vi "GUI_Single Button Pump.vi"() -> ()   [LabVIEW 2011] (continued)
        w1447 = T32[] [enum."Is the LB Roughing Pipe at Atmospheric Pressure?", enum."Is the LB Roughing Manifold at Atmospheric Pressure"] items=["No Action", "Is EC GPM Mode ON?", "Is EC GPM Mode Off?", "Is EC GVM Mode ON?", "Is EC GVM Off?", "Is  EC GPM or GVM Mode ON?", "Is LB GPM Mode ON?", "Is LB GPM Mode Off?", "Is LB GVM Mode ON?", "Is LB GVM Mode Off?", "Is  LB GPM or GVM Mode ON?", "Is M123 Turbo Gate Valve Opened? ", "Is M123 Turbo Gate Valve Closed?", "Is OAP Turbo Gate Valve Opened?", "Is OAP Turbo Gate Valve Closed?", "Is BTLTurbo Gate Valve Opened?", "Is BTL Turbo Gate Valve Closed?", "Is TARGET Turbo Gate Valve 1Opened?", "Is TARGET1 Turbo Gate Valve Closed?", "Is TARGET Turbo Gate Valve 2 Opened?", "Is TAREGT2 Turbo Gate Valve Closed?", "Is BTL2 Turbo Gate Valve Opened?", "Is BTL2 Turbo Gate Valve Closed?", "Is HPD Turbo Gate Valve Opened?", "Is HPD Turbo Gate Valve Closed?", "Is COMP to M123 gate Valve Opened?", "Is COMP to M123 Valve Closed?", "Is HPBD Gate Valve Opened?", "Is HPBD Gate Valve Closed?", "Is M123 to OAP gate valve opened?", "Is M123 to OAP gate valve closed?", "Is OAP to BLT gate valve opened?", "Is OAP to BTL Gate Valve Closed?", "Is BLT to TARGET gate valve opened?", "Is BTL to TARGET Gate Valve Closed?", "Is TARGET to BLT2 gate valve opened?", "Is TARGET to BTL2 Gate Valve Closed?", "Is BLT2 to HPD gate valve opened?", "Is BTL2 to HPD Gate Valve Closed?", "Is COMP at Atmospheric Pressure?", "Is M123 at Atmospheric Pressure?", "Is BeamDump at Atmospheric Pressure?", "Is OAP at Atmospheric Pressure?", "Is BLT at Atmospheric Pressure", "Is TARGET at Atmospheric Pressure?", "Is BLT2 at Atmospheric Pressure?", "Is HPD at Atmospheric Pressure?", "Is the EC Roughing Pump ON?", "Is the EC Roughing Pump OFF?", "Does the EC Roughing Pump have a fault?", "Is the LB Roughing Pump ON?", "Is the LB Roughing Pump Off?", "Does the LB Roughing Pump have a fault?", "Is the EC Backing Pump ON?", "Is the EC Backing Pump OFF?", "Is the LB Backing Pump ON?", "Is the LB Backing Pump OFF?", "Does the EC Backing Pump have a fault?", "Does the LB Backing Pump have a fault?", "Is the EC Backing Pipe at Atmospheric Pressure", "Is the LB Backing Pipe at Atmospheric Pressure", "Is the EC Backing Manifold at Atmospheric Pressure", "s the LB Backing Manifold at Atmospheric Pressure?", "Is the EC Roughing Pipe at Atmospheric Pressure", "Is the LB Roughing Pipe at Atmospheric Pressure?", "Is the EC Roughing Manifold at Atmospheric Pressure", "Is the LB Roughing Manifold at Atmospheric Pressure", "Is LB Backing Manifold Valve Opened?", "Is EC Backing Manifold Valve Opened?", "Is LB Roughing Manifold Valve Opened?", "Is EC Roughing Manifold Valve Opened?", "Is COMP Roughing Valve Opened?", "Is M123 Roughing Valve Opened?", "Is M123 Roughing Valve Closed?", "Is OAP Roughing Valve Opened?", "Is OAP Roughing Valve Closed?", "Is HPBD Roughing Valve Opened?", "Is HPBD Roughing Valve Closed?", "Is BTL Roughing Valve Opened?", "Is BTL Roughing Valve Closed?", "Is TARGET Roughing Valve Opened?", "Is TARGET Roughing Valve Closed?", "Is BTL2 Roughing Valve Opened?", "Is BTL2 Roughing Valve Closed?", "Is HPD Roughing Valve Opened?", "Is HPD Roughing Valve Closed?", "Is COMP Turbo Backing Valve Opened?", "Is M123 Turbo Backing Valve Opened", "Is HPBD Turbo Backing Valve Opened?", "Is OAP Turbo Backing Valve Opened?", "Is BTL Turbo Backing Valve Opened?", "Is TARGET1 Turbo Backing Valve Opened?", "Is TARGET2 Turbo Backing Valve Opened?", "Is BTL2 Turbo Backing Valve Opened?", "Is HPD Turbo Backing Valve Opened?", "Is M123 Backing at MID-VAC?", "Is OAP Backing at MID-VAC?", "Is TARGET1 Backing at MID-VAC?", "Is TARGET2 Backing at MID-VAC?", "Is BTL Backing at MID-VAC?", "Is BTL2 Backing at MID-VAC?", "Is HPD Backing at MID-VAC?", "Is M123 Turbo in Normal Operation", "Is COMP Turbo in Normal Operation", "Is OAP Turbo in Normal Operation", "Is BTL Turbo in Normal Operation", "Is TARGET1 Turbo in Normal Operation", "Is TARGET2 Turbo in Normal Operation", "Is BTL2 Turbo in Normal Operation", "Is HPD Turbo in Normal Operation", "Is M123 at MID-VAC?", "Is OAP at MID-VAC?", "Is COMP at MID-VAC?", "Is BTL at MID-VAC?", "Is TARGET at MID-VAC?", "Is BTL2 at MID-VAC?", "Is HPD at MID-VAC?"]
        # "Event TAG"
        n558 = Unbundle By Name(w1449) -> ("Chamber Selection"=w1448:T21)
        n559 = call "Selection ActionBuilder sections.vi"("EC Query Array"=w1446, "LB Query Array"=w1447, "Chamber Selection"=w1448) -> ("Query Array out"=w1445:T32[])  [unwired: 7 in, 1 out]
        n560 = call "GetAction.vi"("Check Condition"=w1462, "Query Array"=w1445, "input cluster"=w1449, "error in (no error)"=w1464) -> ("Status Array Out"=w1463:string[], "Generate Event?"=w1452:bool, "error out"=w1460:errorcluster)  [unwired: 6 in, 3 out]
        n561 = call "Generate User Event.vi"("Add(t)/Remove(f) Event"=w1452, "error in (no error)"=w1460, "User Event in"=w1461, "Status Array In"=w1463, "Error Codes"=w1462) -> ("error out"=w1459:errorcluster)  [unwired: 5 in, 1 out]
        n562 = Unbundle By Name(w1449) -> ("VI Refnum"=w1454:refnum<vi>)
        n563 = Not A Number/Path/Refnum?(number/path/refnum=w1454) -> (NaN/Path/Refnum?=w1453:bool)
        n564 = case shown="False" w1452 {
          tunnel: ["Main: Open Roughing Manifold Valves" w1480] -> w1450
          tunnel: w1454 -> [w1470 w1479]
          tunnel: w1453 -> [w1471 w1478]
          frame False {
            n565 = case shown="True" w1471 {
              tunnel: w1470 -> [_ w1474]
              frame False {
              }
              frame True {
                n566 = invoke class="VI" method="Abort VI"(reference=w1474) -> (reference out=w1472:refnum<vi>, error out=w1473:errorcluster)  [unwired: 2 in, 1 out]
                n567 = case shown="No Error" w1473 {
                  selector: w1473 -> [w1476 _]
                  tunnel: w1472 -> [w1477 _]
                  frame No Error {
                    n568 = Close Reference(reference=w1477, error in (no error)=w1476) -> (error out=w1475:errorcluster)
                    n569 = invoke on="User Input Panel" class="SubPnl" method="Remove VI"(error in=w1475) -> ()  [unwired: 2 in, 3 out]
                  }
                  frame Error {
                  }
                }
              }
            }
            n570 = call "MID-VAC Timer.vi"("TO sec (Start timer)"=5.0, "Action"=timerAction_typdef."Start Timer") -> ()  [unwired: 9 in, 1 out]
          }
          frame True {
            # "when to is true\nand"
            n571 = case shown="False" w1478 {
              tunnel: w1479 -> [w1484 _]
              tunnel: [w1482 "Main: Check Roughing Manifold Pressure Status"] -> w1480
              frame False {
                n572 = call "FindControlByName_VEPS.vi"("control name"="Op Out", "vi refnum"=w1484) -> ("control refnum"=w1486:refnum<vi>)  [unwired: 2 in, 1 out]
                n573 = property class="Ctl"(reference=w1486) -> ("Value"=w1485:variant)  [unwired: 1 in, 2 out]
                n574 = Variant To Data(type=op_typdef."Idle" ("Op Out"), Variant=w1485) -> (data=w1483:T24)  [unwired: 1 in, 1 out]
                n575 = case shown="\"Idle\", Default" w1483 {
                  tunnel: ["Main: Check Roughing Manifold Pressure Status" "Main: Check Roughing Manifold Pressure Status" "Idle\nMacro: Exit"] -> w1482
                  frame "Idle", Default {
                    n576 = call "MID-VAC Timer.vi"("TO sec (Start timer)"=30.0, "Action"=timerAction_typdef."Start Timer") -> ()  [unwired: 9 in, 1 out]
                  }
                  frame "Continue to Wait" {
                    # "Continue to wait. Reset Timer"
                    n577 = call "MID-VAC Timer.vi"("TO sec (Start timer)"=30.0, "Action"=timerAction_typdef."Start Timer") -> ()  [unwired: 9 in, 1 out]
                  }
                  frame "Exit" {
                  }
                }
              }
              frame True {
              }
            }
          }
        }
        n578 = call "MID-VAC Timer.vi"("Action"=timerAction_typdef."Timer Running") -> ("TO"=w1457:bool)  [unwired: 10 in]
        n579 = And(x=w1452, y=w1457) -> (x .and. y?=w1456:bool)
        n580 = call "Generate TO event.vi"("Boolean"=w1456, "message"="Roughing Pipe and Manifold are not Vented\nPlease perform corrective action\n and click on continue.\nClick Exit to abort GPM", "User Event in"=w1451) -> ()  [unwired: 9 in]
        n581 = call <vilib>:"Add State(s) to Queue__jki_lib_state_machine.vi"("State(s) in (\"\")"=w1466, "State(s) at Back (\"\")"=w1450) -> ("States Out"=w1465:string)  [unwired: 13 in]
      }
      frame "Main: Open Roughing Manifold Valves" {
        # "Open Backing Valves on both systems"
        n582 = Unbundle By Name(w1497) -> ("Debug Mode?"=w1496:bool)
        n583 = case shown="False" w1496 {
          tunnel: w1503 -> [w1513 w1518]
          tunnel: [w1510 w1518] -> w1501
          tunnel: w1497 -> [w1508 _]
          frame False {
            w1507 = T33[] [enum."Open LB Roughing Valve"] items=["No Action", "Set GPM Mode LB", "EXIT GPM Mode LB", "Set GPM Mode EC", "EXIT GPM Mode EC", "Set GVM mode LB", "Set GVM Mode EC", "Open LB Backing Valve", "Open EC Backing Valve", "Open EC Roughing Valve", "Open LB Roughing Valve", "Open M123 Roughing Valve", "Close M123 Roughing Valve", "Open Compressor Roughing Valve", "Close Compressor Roughing Valve", "Open BeamDump Roughing Valve", "Close BeamDump Roughing Valve", "Open OAP Roughing Valve", "Close OAP Roughing Valve", "Open BTL Roughing Valve", "Close BTL Roughing Valve", "Open Target Roughing Valve", "Close Target Roughing Valve", "Open BTL2 Roughing Valve", "Close BTL2 Roughing Valve", "Open HPD Roughing Valve", "Close HPD Roughing Valve", "LB Start Roughing Pump ", "EC Start Roughing Pump", "Open COMP Turbo Backing Valve", "Open M123 Turbo Backing Valve", "Open OAP Turbo Backing Valve", "Open HPBD Turbo Backing Valve", "Open BLT Turbo Backing Valve", "Open TARGET1 Turbo Backing Valve", "Open TARGET2 Turbo Backing Valve", "Open BLT2 Turbo Backing Valve", "Open HPD Turbo Backing Valve", "LB Start Turbo Backing Pump", "EC Start Turbo Backing Pump", "Start COMP Turbo Pump", "Start M123 Turbo Pump", "Start OAP Turbo Pump", "Start BTL Turbo Pump", "Start TARGET1 Turbo Pump", "Start TARGET2 Turbo Pump", "Start BTL2 Turbo Pump", "Start HPD Turbo Pump", "Open COMP Turbo Gate Valve", "Open M123 Turbo Gate Valve", "Open OAP Turbo Gate Valve", "Open BTL Turbo Gate Valve", "Open TARGET1 Turbo Gate Valve", "Open TARGET2 Turbo Gate Valve", "Open BTL2 Turbo Gate Valve", "Open HPD Turbo Gate Valve"]
            w1506 = T33[] [enum."Open EC Roughing Valve"] items=["No Action", "Set GPM Mode LB", "EXIT GPM Mode LB", "Set GPM Mode EC", "EXIT GPM Mode EC", "Set GVM mode LB", "Set GVM Mode EC", "Open LB Backing Valve", "Open EC Backing Valve", "Open EC Roughing Valve", "Open LB Roughing Valve", "Open M123 Roughing Valve", "Close M123 Roughing Valve", "Open Compressor Roughing Valve", "Close Compressor Roughing Valve", "Open BeamDump Roughing Valve", "Close BeamDump Roughing Valve", "Open OAP Roughing Valve", "Close OAP Roughing Valve", "Open BTL Roughing Valve", "Close BTL Roughing Valve", "Open Target Roughing Valve", "Close Target Roughing Valve", "Open BTL2 Roughing Valve", "Close BTL2 Roughing Valve", "Open HPD Roughing Valve", "Close HPD Roughing Valve", "LB Start Roughing Pump ", "EC Start Roughing Pump", "Open COMP Turbo Backing Valve", "Open M123 Turbo Backing Valve", "Open OAP Turbo Backing Valve", "Open HPBD Turbo Backing Valve", "Open BLT Turbo Backing Valve", "Open TARGET1 Turbo Backing Valve", "Open TARGET2 Turbo Backing Valve", "Open BLT2 Turbo Backing Valve", "Open HPD Turbo Backing Valve", "LB Start Turbo Backing Pump", "EC Start Turbo Backing Pump", "Start COMP Turbo Pump", "Start M123 Turbo Pump", "Start OAP Turbo Pump", "Start BTL Turbo Pump", "Start TARGET1 Turbo Pump", "Start TARGET2 Turbo Pump", "Start BTL2 Turbo Pump", "Start HPD Turbo Pump", "Open COMP Turbo Gate Valve", "Open M123 Turbo Gate Valve", "Open OAP Turbo Gate Valve", "Open BTL Turbo Gate Valve", "Open TARGET1 Turbo Gate Valve", "Open TARGET2 Turbo Gate Valve", "Open BTL2 Turbo Gate Valve", "Open HPD Turbo Gate Valve"]
            n584 = Unbundle By Name(w1508) -> ("Chamber Selection"=w1509:T21)
            n585 = call "Selection ActionBuilder sections.vi"("EC Command Array"=w1506, "Chamber Selection"=w1509, "LB Command Array"=w1507) -> ("Command Array out"=w1505:T33[])  [unwired: 7 in, 1 out]
            n586 = Unbundle By Name(w1508) -> ("TCPConnection.Command TCP Connection EC"=w1514:refnum<k5>)
            n587 = Unbundle By Name(w1508) -> ("TCPConnection.Command TCP Connection LB"=w1516:refnum<k5>)
            n588 = call "Build Command.vi"("Command Array in"=w1505, "input cluster"=w1508) -> ("output EC Command cluster"=w1515:T34, "output LB Command cluster"=w1517:T34)  [unwired: 8 in]
            n589 = call "Send Command LB.vi"("error in (no error)"=w1513, "output LB Command cluster"=w1517, "TCP Network Connection in"=w1516) -> ("error out"=w1511:errorcluster)  [unwired: 8 in]
            n590 = call "Send Command EC.vi"("error in (no error)"=w1513, "output EC Command cluster"=w1515, "TCP Network Connection in"=w1514) -> ("error out"=w1512:errorcluster)  [unwired: 8 in]
            n591 = Merge Errors(w1511, w1512) -> (w1510:errorcluster)
          }
          frame True {
          }
        }
        n592 = call "Reset Command Clusters.vi"("error in (no error)"=w1501, "input cluster"=w1497) -> ("error out"=w1500:errorcluster, "output cluster"=w1499:T20)  [unwired: 8 in]
        n593 = call <vilib>:"Add State(s) to Queue__jki_lib_state_machine.vi"("State(s) in Front (\"\")"="Main: Check Roughing Manifold Valve Status", "State(s) in (\"\")"=w1498) -> ("States Out"=w1504:string)  [unwired: 13 in]
      }
      frame "Main: Check Roughing Manifold Valve Status" {
        w1521 = T32[] [enum."Is EC Roughing Manifold Valve Opened?"] items=["No Action", "Is EC GPM Mode ON?", "Is EC GPM Mode Off?", "Is EC GVM Mode ON?", "Is EC GVM Off?", "Is  EC GPM or GVM Mode ON?", "Is LB GPM Mode ON?", "Is LB GPM Mode Off?", "Is LB GVM Mode ON?", "Is LB GVM Mode Off?", "Is  LB GPM or GVM Mode ON?", "Is M123 Turbo Gate Valve Opened? ", "Is M123 Turbo Gate Valve Closed?", "Is OAP Turbo Gate Valve Opened?", "Is OAP Turbo Gate Valve Closed?", "Is BTLTurbo Gate Valve Opened?", "Is BTL Turbo Gate Valve Closed?", "Is TARGET Turbo Gate Valve 1Opened?", "Is TARGET1 Turbo Gate Valve Closed?", "Is TARGET Turbo Gate Valve 2 Opened?", "Is TAREGT2 Turbo Gate Valve Closed?", "Is BTL2 Turbo Gate Valve Opened?", "Is BTL2 Turbo Gate Valve Closed?", "Is HPD Turbo Gate Valve Opened?", "Is HPD Turbo Gate Valve Closed?", "Is COMP to M123 gate Valve Opened?", "Is COMP to M123 Valve Closed?", "Is HPBD Gate Valve Opened?", "Is HPBD Gate Valve Closed?", "Is M123 to OAP gate valve opened?", "Is M123 to OAP gate valve closed?", "Is OAP to BLT gate valve opened?", "Is OAP to BTL Gate Valve Closed?", "Is BLT to TARGET gate valve opened?", "Is BTL to TARGET Gate Valve Closed?", "Is TARGET to BLT2 gate valve opened?", "Is TARGET to BTL2 Gate Valve Closed?", "Is BLT2 to HPD gate valve opened?", "Is BTL2 to HPD Gate Valve Closed?", "Is COMP at Atmospheric Pressure?", "Is M123 at Atmospheric Pressure?", "Is BeamDump at Atmospheric Pressure?", "Is OAP at Atmospheric Pressure?", "Is BLT at Atmospheric Pressure", "Is TARGET at Atmospheric Pressure?", "Is BLT2 at Atmospheric Pressure?", "Is HPD at Atmospheric Pressure?", "Is the EC Roughing Pump ON?", "Is the EC Roughing Pump OFF?", "Does the EC Roughing Pump have a fault?", "Is the LB Roughing Pump ON?", "Is the LB Roughing Pump Off?", "Does the LB Roughing Pump have a fault?", "Is the EC Backing Pump ON?", "Is the EC Backing Pump OFF?", "Is the LB Backing Pump ON?", "Is the LB Backing Pump OFF?", "Does the EC Backing Pump have a fault?", "Does the LB Backing Pump have a fault?", "Is the EC Backing Pipe at Atmospheric Pressure", "Is the LB Backing Pipe at Atmospheric Pressure", "Is the EC Backing Manifold at Atmospheric Pressure", "s the LB Backing Manifold at Atmospheric Pressure?", "Is the EC Roughing Pipe at Atmospheric Pressure", "Is the LB Roughing Pipe at Atmospheric Pressure?", "Is the EC Roughing Manifold at Atmospheric Pressure", "Is the LB Roughing Manifold at Atmospheric Pressure", "Is LB Backing Manifold Valve Opened?", "Is EC Backing Manifold Valve Opened?", "Is LB Roughing Manifold Valve Opened?", "Is EC Roughing Manifold Valve Opened?", "Is COMP Roughing Valve Opened?", "Is M123 Roughing Valve Opened?", "Is M123 Roughing Valve Closed?", "Is OAP Roughing Valve Opened?", "Is OAP Roughing Valve Closed?", "Is HPBD Roughing Valve Opened?", "Is HPBD Roughing Valve Closed?", "Is BTL Roughing Valve Opened?", "Is BTL Roughing Valve Closed?", "Is TARGET Roughing Valve Opened?", "Is TARGET Roughing Valve Closed?", "Is BTL2 Roughing Valve Opened?", "Is BTL2 Roughing Valve Closed?", "Is HPD Roughing Valve Opened?", "Is HPD Roughing Valve Closed?", "Is COMP Turbo Backing Valve Opened?", "Is M123 Turbo Backing Valve Opened", "Is HPBD Turbo Backing Valve Opened?", "Is OAP Turbo Backing Valve Opened?", "Is BTL Turbo Backing Valve Opened?", "Is TARGET1 Turbo Backing Valve Opened?", "Is TARGET2 Turbo Backing Valve Opened?", "Is BTL2 Turbo Backing Valve Opened?", "Is HPD Turbo Backing Valve Opened?", "Is M123 Backing at MID-VAC?", "Is OAP Backing at MID-VAC?", "Is TARGET1 Backing at MID-VAC?", "Is TARGET2 Backing at MID-VAC?", "Is BTL Backing at MID-VAC?", "Is BTL2 Backing at MID-VAC?", "Is HPD Backing at MID-VAC?", "Is M123 Turbo in Normal Operation", "Is COMP Turbo in Normal Operation", "Is OAP Turbo in Normal Operation", "Is BTL Turbo in Normal Operation", "Is TARGET1 Turbo in Normal Operation", "Is TARGET2 Turbo in Normal Operation", "Is BTL2 Turbo in Normal Operation", "Is HPD Turbo in Normal Operation", "Is M123 at MID-VAC?", "Is OAP at MID-VAC?", "Is COMP at MID-VAC?", "Is BTL at MID-VAC?", "Is TARGET at MID-VAC?", "Is BTL2 at MID-VAC?", "Is HPD at MID-VAC?"]
        w1536 = Error_codes."010-Roughing Valve Status" ("Error Codes")
        w1520 = T32[] [enum."Is LB Roughing Manifold Valve Opened?"] items=["No Action", "Is EC GPM Mode ON?", "Is EC GPM Mode Off?", "Is EC GVM Mode ON?", "Is EC GVM Off?", "Is  EC GPM or GVM Mode ON?", "Is LB GPM Mode ON?", "Is LB GPM Mode Off?", "Is LB GVM Mode ON?", "Is LB GVM Mode Off?", "Is  LB GPM or GVM Mode ON?", "Is M123 Turbo Gate Valve Opened? ", "Is M123 Turbo Gate Valve Closed?", "Is OAP Turbo Gate Valve Opened?", "Is OAP Turbo Gate Valve Closed?", "Is BTLTurbo Gate Valve Opened?", "Is BTL Turbo Gate Valve Closed?", "Is TARGET Turbo Gate Valve 1Opened?", "Is TARGET1 Turbo Gate Valve Closed?", "Is TARGET Turbo Gate Valve 2 Opened?", "Is TAREGT2 Turbo Gate Valve Closed?", "Is BTL2 Turbo Gate Valve Opened?", "Is BTL2 Turbo Gate Valve Closed?", "Is HPD Turbo Gate Valve Opened?", "Is HPD Turbo Gate Valve Closed?", "Is COMP to M123 gate Valve Opened?", "Is COMP to M123 Valve Closed?", "Is HPBD Gate Valve Opened?", "Is HPBD Gate Valve Closed?", "Is M123 to OAP gate valve opened?", "Is M123 to OAP gate valve closed?", "Is OAP to BLT gate valve opened?", "Is OAP to BTL Gate Valve Closed?", "Is BLT to TARGET gate valve opened?", "Is BTL to TARGET Gate Valve Closed?", "Is TARGET to BLT2 gate valve opened?", "Is TARGET to BTL2 Gate Valve Closed?", "Is BLT2 to HPD gate valve opened?", "Is BTL2 to HPD Gate Valve Closed?", "Is COMP at Atmospheric Pressure?", "Is M123 at Atmospheric Pressure?", "Is BeamDump at Atmospheric Pressure?", "Is OAP at Atmospheric Pressure?", "Is BLT at Atmospheric Pressure", "Is TARGET at Atmospheric Pressure?", "Is BLT2 at Atmospheric Pressure?", "Is HPD at Atmospheric Pressure?", "Is the EC Roughing Pump ON?", "Is the EC Roughing Pump OFF?", "Does the EC Roughing Pump have a fault?", "Is the LB Roughing Pump ON?", "Is the LB Roughing Pump Off?", "Does the LB Roughing Pump have a fault?", "Is the EC Backing Pump ON?", "Is the EC Backing Pump OFF?", "Is the LB Backing Pump ON?", "Is the LB Backing Pump OFF?", "Does the EC Backing Pump have a fault?", "Does the LB Backing Pump have a fault?", "Is the EC Backing Pipe at Atmospheric Pressure", "Is the LB Backing Pipe at Atmospheric Pressure", "Is the EC Backing Manifold at Atmospheric Pressure", "s the LB Backing Manifold at Atmospheric Pressure?", "Is the EC Roughing Pipe at Atmospheric Pressure", "Is the LB Roughing Pipe at Atmospheric Pressure?", "Is the EC Roughing Manifold at Atmospheric Pressure", "Is the LB Roughing Manifold at Atmospheric Pressure", "Is LB Backing Manifold Valve Opened?", "Is EC Backing Manifold Valve Opened?", "Is LB Roughing Manifold Valve Opened?", "Is EC Roughing Manifold Valve Opened?", "Is COMP Roughing Valve Opened?", "Is M123 Roughing Valve Opened?", "Is M123 Roughing Valve Closed?", "Is OAP Roughing Valve Opened?", "Is OAP Roughing Valve Closed?", "Is HPBD Roughing Valve Opened?", "Is HPBD Roughing Valve Closed?", "Is BTL Roughing Valve Opened?", "Is BTL Roughing Valve Closed?", "Is TARGET Roughing Valve Opened?", "Is TARGET Roughing Valve Closed?", "Is BTL2 Roughing Valve Opened?", "Is BTL2 Roughing Valve Closed?", "Is HPD Roughing Valve Opened?", "Is HPD Roughing Valve Closed?", "Is COMP Turbo Backing Valve Opened?", "Is M123 Turbo Backing Valve Opened", "Is HPBD Turbo Backing Valve Opened?", "Is OAP Turbo Backing Valve Opened?", "Is BTL Turbo Backing Valve Opened?", "Is TARGET1 Turbo Backing Valve Opened?", "Is TARGET2 Turbo Backing Valve Opened?", "Is BTL2 Turbo Backing Valve Opened?", "Is HPD Turbo Backing Valve Opened?", "Is M123 Backing at MID-VAC?", "Is OAP Backing at MID-VAC?", "Is TARGET1 Backing at MID-VAC?", "Is TARGET2 Backing at MID-VAC?", "Is BTL Backing at MID-VAC?", "Is BTL2 Backing at MID-VAC?", "Is HPD Backing at MID-VAC?", "Is M123 Turbo in Normal Operation", "Is COMP Turbo in Normal Operation", "Is OAP Turbo in Normal Operation", "Is BTL Turbo in Normal Operation", "Is TARGET1 Turbo in Normal Operation", "Is TARGET2 Turbo in Normal Operation", "Is BTL2 Turbo in Normal Operation", "Is HPD Turbo in Normal Operation", "Is M123 at MID-VAC?", "Is OAP at MID-VAC?", "Is COMP at MID-VAC?", "Is BTL at MID-VAC?", "Is TARGET at MID-VAC?", "Is BTL2 at MID-VAC?", "Is HPD at MID-VAC?"]
        # "Event TAG"
        n594 = Unbundle By Name(w1522) -> ("Chamber Selection"=w1523:T21)
        n595 = call "Selection ActionBuilder sections.vi"("EC Query Array"=w1521, "LB Query Array"=w1520, "Chamber Selection"=w1523) -> ("Query Array out"=w1519:T32[])  [unwired: 7 in, 1 out]
        n596 = call "GetAction.vi"("Check Condition"=w1536, "Query Array"=w1519, "input cluster"=w1522, "error in (no error)"=w1538) -> ("Status Array Out"=w1537:string[], "Generate Event?"=w1526:bool, "error out"=w1534:errorcluster)  [unwired: 6 in, 3 out]
        n597 = call "Generate User Event.vi"("Add(t)/Remove(f) Event"=w1526, "error in (no error)"=w1534, "User Event in"=w1535, "Status Array In"=w1537, "Error Codes"=w1536) -> ("error out"=w1533:errorcluster)  [unwired: 5 in, 1 out]
        n598 = Unbundle By Name(w1522) -> ("VI Refnum"=w1528:refnum<vi>)
        n599 = Not A Number/Path/Refnum?(number/path/refnum=w1528) -> (NaN/Path/Refnum?=w1527:bool)
        n600 = case shown="False" w1526 {
          tunnel: ["Macro: Roughing Valve Precheck Selection" w1554] -> w1524
          tunnel: w1528 -> [w1544 w1553]
          tunnel: w1527 -> [w1545 w1552]
          frame False {
            # "Proceed to next step"
            n601 = case shown="False" w1545 {
              tunnel: w1544 -> [_ w1548]
              frame False {
              }
              frame True {
                n602 = invoke class="VI" method="Abort VI"(reference=w1548) -> (reference out=w1546:refnum<vi>, error out=w1547:errorcluster)  [unwired: 2 in, 1 out]
                n603 = case shown="No Error" w1547 {
                  selector: w1547 -> [w1550 _]
                  tunnel: w1546 -> [w1551 _]
                  frame No Error {
                    n604 = Close Reference(reference=w1551, error in (no error)=w1550) -> (error out=w1549:errorcluster)
                    n605 = invoke on="User Input Panel" class="SubPnl" method="Remove VI"(error in=w1549) -> ()  [unwired: 2 in, 3 out]
                  }
                  frame Error {
                  }
                }
              }
            }
            n606 = call "MID-VAC Timer.vi"("TO sec (Start timer)"=5.0, "Action"=timerAction_typdef."Start Timer") -> ()  [unwired: 9 in, 1 out]
          }
          frame True {
            # "when to is true\nand"
            n607 = case shown="False" w1552 {
              tunnel: w1553 -> [w1558 _]
              tunnel: [w1556 "Main: Check Roughing Manifold Valve Status"] -> w1554
              frame False {
                n608 = call "FindControlByName_VEPS.vi"("control name"="Op Out", "vi refnum"=w1558) -> ("control refnum"=w1560:refnum<vi>)  [unwired: 2 in, 1 out]
                n609 = property class="Ctl"(reference=w1560) -> ("Value"=w1559:variant)  [unwired: 1 in, 2 out]
                n610 = Variant To Data(type=op_typdef."Idle" ("Op Out"), Variant=w1559) -> (data=w1557:T24)  [unwired: 1 in, 1 out]
                n611 = case shown="\"Idle\", Default" w1557 {
                  tunnel: ["Main: Check Roughing Manifold Valve Status" "Main: Check Roughing Manifold Valve Status" "Idle\nMacro: Exit"] -> w1556
                  frame "Idle", Default {
                    n612 = call "MID-VAC Timer.vi"("TO sec (Start timer)"=30.0, "Action"=timerAction_typdef."Start Timer") -> ()  [unwired: 9 in, 1 out]
                  }
                  frame "Continue to Wait" {
                    # "Continue to wait. Reset Timer"
                    n613 = call "MID-VAC Timer.vi"("TO sec (Start timer)"=30.0, "Action"=timerAction_typdef."Start Timer") -> ()  [unwired: 9 in, 1 out]
                  }
                  frame "Exit" {
                  }
                }
              }
              frame True {
              }
            }
          }
        }
        n614 = call "MID-VAC Timer.vi"("Action"=timerAction_typdef."Timer Running") -> ("TO"=w1531:bool)  [unwired: 10 in]
        n615 = And(x=w1526, y=w1531) -> (x .and. y?=w1530:bool)
        n616 = call <vilib>:"Add State(s) to Queue__jki_lib_state_machine.vi"("State(s) in Front (\"\")"=w1524, "State(s) in (\"\")"=w1540) -> ("States Out"=w1539:string)  [unwired: 13 in]
        n617 = call "Generate TO event.vi"("Boolean"=w1530, "message"="Roughing Manifold Valve is NOT open.\nPlease perform corrective action\nClick on continue to wait for 30 seconds.\nClick Exit to abort GPM", "User Event in"=w1525) -> ()  [unwired: 9 in]
      }
      frame "---------- Main: Roughing Valves----------" {
      }
      frame "Macro: Roughing Valve Precheck Selection" {
        # "3. Start Roughing pumps after all prechecks for roughing valves\nhave been completed and the roughing valves for selected chambers\nare opened."
        # "1. Check if only some chambers are selected"
        n618 = Unbundle By Name(w1578) -> ("Chamber Selection"=w1577:T21, "Isolate HPBD"=w1580:bool, "GPM Mode"=w1582:T1)
        n619 = Equal?(x=w1582, y=GPM_Mode_typdef."Complete Global Pump Mode" ("GPM Mode")) -> (x = y?=w1579:bool)
        n620 = case shown="True" w1579 {
          tunnel: [w1586 w1590] -> w1574
          tunnel: w1580 -> [w1588 w1589]
          tunnel: w1578 -> [_ _]
          tunnel: w1577 -> [w1587 _]
          frame False {
            # "2. All chambers not selected. Roughing Valve checks \nwill be performed only on selected chambers"
            n621 = call "Roughing Valve Precheck Selection.vi"("Isolate HPBD"=w1588, "Chamber Selection"=w1587) -> ("States Out"=w1586:string)  [unwired: 9 in]
          }
          frame True {
            # "2. All chambers are selected."
            n622 = case shown="False" w1589 {
              tunnel: ["Main: Roughing Valve Precheck>>M123\nMain: Open Roughing Valve>>M123\nMain: Check Roughing Valve Status>>M123\nMain: Roughing Valve Precheck>>HPBD\nMain: Open Roughing Valve>>HPBD\nMain: Check Roughing Valve Status>>HPBD\nMain: Roughing Valve Precheck>>OAP\nMain: Open Roughing Valve>>OAP\nMain: Check Roughing Valve Status>>OAP\nMain: Roughing Valve Precheck>>BTL\nMain: Open Roughing Valve>>BTL\nMain: Check Roughing Valve Status>>BTL\nMain: Roughing Valve Precheck>>TARGET\nMain: Open Roughing Valve>>TARGET\nMain: Check Roughing Valve Status>>TARGET\nMain: Roughing Valve Precheck>>BTL2\nMain: Open Roughing Valve>>BTL2\nMain: Check Roughing Valve Status>>BTL2\nMain: Roughing Valve Precheck>>HPD\nMain: Open Roughing Valve>>HPD\nMain: Check Roughing Valve Status>>HPD" "Main: Roughing Valve Precheck>>M123\nMain: Open Roughing Valve>>M123\nMain: Check Roughing Valve Status>>M123\nMain: Roughing Valve Precheck>>OAP\nMain: Open Roughing Valve>>OAP\nMain: Check Roughing Valve Status>>OAP\nMain: Roughing Valve Precheck>>BTL\nMain: Open Roughing Valve>>BTL\nMain: Check Roughing Valve Status>>BTL\nMain: Roughing Valve Precheck>>TARGET\nMain: Open Roughing Valve>>TARGET\nMain: Check Roughing Valve Status>>TARGET\nMain: Roughing Valve Precheck>>BTL2\nMain: Open Roughing Valve>>BTL2\nMain: Check Roughing Valve Status>>BTL2\nMain: Roughing Valve Precheck>>HPD\nMain: Open Roughing Valve>>HPD\nMain: Check Roughing Valve Status>>HPD"] -> w1590
              frame False {
                # "HPBD is NOT Isolated"
              }
              frame True {
                # "HPBD is Isolated"
              }
            }
          }
        }
        n623 = Concatenate Strings(w1574, "\n", "Main: Start Roughing Pumps" ("string")) -> (w1573:string)
        n624 = call <vilib>:"Add State(s) to Queue__jki_lib_state_machine.vi"("State(s) in Front (\"\")"=w1573, "State(s) in (\"\")"=w1585) -> ("States Out"=w1584:string)  [unwired: 13 in]
      }
      frame "Main: Roughing Valve Precheck" {
        w1606 = Error_codes."004-Check Chamber Pressures" ("Error Codes")
        n625 = case shown="\"BTL2\"" w1596 {
          tunnel: [_ w1630 w1631 w1632 w1633 w1634 w1635 w1636] -> w1609
          frame "False", Default {
          }
          frame "M123" {
            w1630 = T32[] [enum."Is M123 at Atmospheric Pressure?", enum."Is the LB Roughing Manifold at Atmospheric Pressure"] items=["No Action", "Is EC GPM Mode ON?", "Is EC GPM Mode Off?", "Is EC GVM Mode ON?", "Is EC GVM Off?", "Is  EC GPM or GVM Mode ON?", "Is LB GPM Mode ON?", "Is LB GPM Mode Off?", "Is LB GVM Mode ON?", "Is LB GVM Mode Off?", "Is  LB GPM or GVM Mode ON?", "Is M123 Turbo Gate Valve Opened? ", "Is M123 Turbo Gate Valve Closed?", "Is OAP Turbo Gate Valve Opened?", "Is OAP Turbo Gate Valve Closed?", "Is BTLTurbo Gate Valve Opened?", "Is BTL Turbo Gate Valve Closed?", "Is TARGET Turbo Gate Valve 1Opened?", "Is TARGET1 Turbo Gate Valve Closed?", "Is TARGET Turbo Gate Valve 2 Opened?", "Is TAREGT2 Turbo Gate Valve Closed?", "Is BTL2 Turbo Gate Valve Opened?", "Is BTL2 Turbo Gate Valve Closed?", "Is HPD Turbo Gate Valve Opened?", "Is HPD Turbo Gate Valve Closed?", "Is COMP to M123 gate Valve Opened?", "Is COMP to M123 Valve Closed?", "Is HPBD Gate Valve Opened?", "Is HPBD Gate Valve Closed?", "Is M123 to OAP gate valve opened?", "Is M123 to OAP gate valve closed?", "Is OAP to BLT gate valve opened?", "Is OAP to BTL Gate Valve Closed?", "Is BLT to TARGET gate valve opened?", "Is BTL to TARGET Gate Valve Closed?", "Is TARGET to BLT2 gate valve opened?", "Is TARGET to BTL2 Gate Valve Closed?", "Is BLT2 to HPD gate valve opened?", "Is BTL2 to HPD Gate Valve Closed?", "Is COMP at Atmospheric Pressure?", "Is M123 at Atmospheric Pressure?", "Is BeamDump at Atmospheric Pressure?", "Is OAP at Atmospheric Pressure?", "Is BLT at Atmospheric Pressure", "Is TARGET at Atmospheric Pressure?", "Is BLT2 at Atmospheric Pressure?", "Is HPD at Atmospheric Pressure?", "Is the EC Roughing Pump ON?", "Is the EC Roughing Pump OFF?", "Does the EC Roughing Pump have a fault?", "Is the LB Roughing Pump ON?", "Is the LB Roughing Pump Off?", "Does the LB Roughing Pump have a fault?", "Is the EC Backing Pump ON?", "Is the EC Backing Pump OFF?", "Is the LB Backing Pump ON?", "Is the LB Backing Pump OFF?", "Does the EC Backing Pump have a fault?", "Does the LB Backing Pump have a fault?", "Is the EC Backing Pipe at Atmospheric Pressure", "Is the LB Backing Pipe at Atmospheric Pressure", "Is the EC Backing Manifold at Atmospheric Pressure", "s the LB Backing Manifold at Atmospheric Pressure?", "Is the EC Roughing Pipe at Atmospheric Pressure", "Is the LB Roughing Pipe at Atmospheric Pressure?", "Is the EC Roughing Manifold at Atmospheric Pressure", "Is the LB Roughing Manifold at Atmospheric Pressure", "Is LB Backing Manifold Valve Opened?", "Is EC Backing Manifold Valve Opened?", "Is LB Roughing Manifold Valve Opened?", "Is EC Roughing Manifold Valve Opened?", "Is COMP Roughing Valve Opened?", "Is M123 Roughing Valve Opened?", "Is M123 Roughing Valve Closed?", "Is OAP Roughing Valve Opened?", "Is OAP Roughing Valve Closed?", "Is HPBD Roughing Valve Opened?", "Is HPBD Roughing Valve Closed?", "Is BTL Roughing Valve Opened?", "Is BTL Roughing Valve Closed?", "Is TARGET Roughing Valve Opened?", "Is TARGET Roughing Valve Closed?", "Is BTL2 Roughing Valve Opened?", "Is BTL2 Roughing Valve Closed?", "Is HPD Roughing Valve Opened?", "Is HPD Roughing Valve Closed?", "Is COMP Turbo Backing Valve Opened?", "Is M123 Turbo Backing Valve Opened", "Is HPBD Turbo Backing Valve Opened?", "Is OAP Turbo Backing Valve Opened?", "Is BTL Turbo Backing Valve Opened?", "Is TARGET1 Turbo Backing Valve Opened?", "Is TARGET2 Turbo Backing Valve Opened?", "Is BTL2 Turbo Backing Valve Opened?", "Is HPD Turbo Backing Valve Opened?", "Is M123 Backing at MID-VAC?", "Is OAP Backing at MID-VAC?", "Is TARGET1 Backing at MID-VAC?", "Is TARGET2 Backing at MID-VAC?", "Is BTL Backing at MID-VAC?", "Is BTL2 Backing at MID-VAC?", "Is HPD Backing at MID-VAC?", "Is M123 Turbo in Normal Operation", "Is COMP Turbo in Normal Operation", "Is OAP Turbo in Normal Operation", "Is BTL Turbo in Normal Operation", "Is TARGET1 Turbo in Normal Operation", "Is TARGET2 Turbo in Normal Operation", "Is BTL2 Turbo in Normal Operation", "Is HPD Turbo in Normal Operation", "Is M123 at MID-VAC?", "Is OAP at MID-VAC?", "Is COMP at MID-VAC?", "Is BTL at MID-VAC?", "Is TARGET at MID-VAC?", "Is BTL2 at MID-VAC?", "Is HPD at MID-VAC?"]
          }
          frame "HPBD" {
            w1631 = T32[] [enum."Is BeamDump at Atmospheric Pressure?", enum."Is the LB Roughing Manifold at Atmospheric Pressure"] items=["No Action", "Is EC GPM Mode ON?", "Is EC GPM Mode Off?", "Is EC GVM Mode ON?", "Is EC GVM Off?", "Is  EC GPM or GVM Mode ON?", "Is LB GPM Mode ON?", "Is LB GPM Mode Off?", "Is LB GVM Mode ON?", "Is LB GVM Mode Off?", "Is  LB GPM or GVM Mode ON?", "Is M123 Turbo Gate Valve Opened? ", "Is M123 Turbo Gate Valve Closed?", "Is OAP Turbo Gate Valve Opened?", "Is OAP Turbo Gate Valve Closed?", "Is BTLTurbo Gate Valve Opened?", "Is BTL Turbo Gate Valve Closed?", "Is TARGET Turbo Gate Valve 1Opened?", "Is TARGET1 Turbo Gate Valve Closed?", "Is TARGET Turbo Gate Valve 2 Opened?", "Is TAREGT2 Turbo Gate Valve Closed?", "Is BTL2 Turbo Gate Valve Opened?", "Is BTL2 Turbo Gate Valve Closed?", "Is HPD Turbo Gate Valve Opened?", "Is HPD Turbo Gate Valve Closed?", "Is COMP to M123 gate Valve Opened?", "Is COMP to M123 Valve Closed?", "Is HPBD Gate Valve Opened?", "Is HPBD Gate Valve Closed?", "Is M123 to OAP gate valve opened?", "Is M123 to OAP gate valve closed?", "Is OAP to BLT gate valve opened?", "Is OAP to BTL Gate Valve Closed?", "Is BLT to TARGET gate valve opened?", "Is BTL to TARGET Gate Valve Closed?", "Is TARGET to BLT2 gate valve opened?", "Is TARGET to BTL2 Gate Valve Closed?", "Is BLT2 to HPD gate valve opened?", "Is BTL2 to HPD Gate Valve Closed?", "Is COMP at Atmospheric Pressure?", "Is M123 at Atmospheric Pressure?", "Is BeamDump at Atmospheric Pressure?", "Is OAP at Atmospheric Pressure?", "Is BLT at Atmospheric Pressure", "Is TARGET at Atmospheric Pressure?", "Is BLT2 at Atmospheric Pressure?", "Is HPD at Atmospheric Pressure?", "Is the EC Roughing Pump ON?", "Is the EC Roughing Pump OFF?", "Does the EC Roughing Pump have a fault?", "Is the LB Roughing Pump ON?", "Is the LB Roughing Pump Off?", "Does the LB Roughing Pump have a fault?", "Is the EC Backing Pump ON?", "Is the EC Backing Pump OFF?", "Is the LB Backing Pump ON?", "Is the LB Backing Pump OFF?", "Does the EC Backing Pump have a fault?", "Does the LB Backing Pump have a fault?", "Is the EC Backing Pipe at Atmospheric Pressure", "Is the LB Backing Pipe at Atmospheric Pressure", "Is the EC Backing Manifold at Atmospheric Pressure", "s the LB Backing Manifold at Atmospheric Pressure?", "Is the EC Roughing Pipe at Atmospheric Pressure", "Is the LB Roughing Pipe at Atmospheric Pressure?", "Is the EC Roughing Manifold at Atmospheric Pressure", "Is the LB Roughing Manifold at Atmospheric Pressure", "Is LB Backing Manifold Valve Opened?", "Is EC Backing Manifold Valve Opened?", "Is LB Roughing Manifold Valve Opened?", "Is EC Roughing Manifold Valve Opened?", "Is COMP Roughing Valve Opened?", "Is M123 Roughing Valve Opened?", "Is M123 Roughing Valve Closed?", "Is OAP Roughing Valve Opened?", "Is OAP Roughing Valve Closed?", "Is HPBD Roughing Valve Opened?", "Is HPBD Roughing Valve Closed?", "Is BTL Roughing Valve Opened?", "Is BTL Roughing Valve Closed?", "Is TARGET Roughing Valve Opened?", "Is TARGET Roughing Valve Closed?", "Is BTL2 Roughing Valve Opened?", "Is BTL2 Roughing Valve Closed?", "Is HPD Roughing Valve Opened?", "Is HPD Roughing Valve Closed?", "Is COMP Turbo Backing Valve Opened?", "Is M123 Turbo Backing Valve Opened", "Is HPBD Turbo Backing Valve Opened?", "Is OAP Turbo Backing Valve Opened?", "Is BTL Turbo Backing Valve Opened?", "Is TARGET1 Turbo Backing Valve Opened?", "Is TARGET2 Turbo Backing Valve Opened?", "Is BTL2 Turbo Backing Valve Opened?", "Is HPD Turbo Backing Valve Opened?", "Is M123 Backing at MID-VAC?", "Is OAP Backing at MID-VAC?", "Is TARGET1 Backing at MID-VAC?", "Is TARGET2 Backing at MID-VAC?", "Is BTL Backing at MID-VAC?", "Is BTL2 Backing at MID-VAC?", "Is HPD Backing at MID-VAC?", "Is M123 Turbo in Normal Operation", "Is COMP Turbo in Normal Operation", "Is OAP Turbo in Normal Operation", "Is BTL Turbo in Normal Operation", "Is TARGET1 Turbo in Normal Operation", "Is TARGET2 Turbo in Normal Operation", "Is BTL2 Turbo in Normal Operation", "Is HPD Turbo in Normal Operation", "Is M123 at MID-VAC?", "Is OAP at MID-VAC?", "Is COMP at MID-VAC?", "Is BTL at MID-VAC?", "Is TARGET at MID-VAC?", "Is BTL2 at MID-VAC?", "Is HPD at MID-VAC?"]
          }
          frame "OAP" {
            w1632 = T32[] [enum."Is OAP at Atmospheric Pressure?", enum."Is the LB Roughing Manifold at Atmospheric Pressure"] items=["No Action", "Is EC GPM Mode ON?", "Is EC GPM Mode Off?", "Is EC GVM Mode ON?", "Is EC GVM Off?", "Is  EC GPM or GVM Mode ON?", "Is LB GPM Mode ON?", "Is LB GPM Mode Off?", "Is LB GVM Mode ON?", "Is LB GVM Mode Off?", "Is  LB GPM or GVM Mode ON?", "Is M123 Turbo Gate Valve Opened? ", "Is M123 Turbo Gate Valve Closed?", "Is OAP Turbo Gate Valve Opened?", "Is OAP Turbo Gate Valve Closed?", "Is BTLTurbo Gate Valve Opened?", "Is BTL Turbo Gate Valve Closed?", "Is TARGET Turbo Gate Valve 1Opened?", "Is TARGET1 Turbo Gate Valve Closed?", "Is TARGET Turbo Gate Valve 2 Opened?", "Is TAREGT2 Turbo Gate Valve Closed?", "Is BTL2 Turbo Gate Valve Opened?", "Is BTL2 Turbo Gate Valve Closed?", "Is HPD Turbo Gate Valve Opened?", "Is HPD Turbo Gate Valve Closed?", "Is COMP to M123 gate Valve Opened?", "Is COMP to M123 Valve Closed?", "Is HPBD Gate Valve Opened?", "Is HPBD Gate Valve Closed?", "Is M123 to OAP gate valve opened?", "Is M123 to OAP gate valve closed?", "Is OAP to BLT gate valve opened?", "Is OAP to BTL Gate Valve Closed?", "Is BLT to TARGET gate valve opened?", "Is BTL to TARGET Gate Valve Closed?", "Is TARGET to BLT2 gate valve opened?", "Is TARGET to BTL2 Gate Valve Closed?", "Is BLT2 to HPD gate valve opened?", "Is BTL2 to HPD Gate Valve Closed?", "Is COMP at Atmospheric Pressure?", "Is M123 at Atmospheric Pressure?", "Is BeamDump at Atmospheric Pressure?", "Is OAP at Atmospheric Pressure?", "Is BLT at Atmospheric Pressure", "Is TARGET at Atmospheric Pressure?", "Is BLT2 at Atmospheric Pressure?", "Is HPD at Atmospheric Pressure?", "Is the EC Roughing Pump ON?", "Is the EC Roughing Pump OFF?", "Does the EC Roughing Pump have a fault?", "Is the LB Roughing Pump ON?", "Is the LB Roughing Pump Off?", "Does the LB Roughing Pump have a fault?", "Is the EC Backing Pump ON?", "Is the EC Backing Pump OFF?", "Is the LB Backing Pump ON?", "Is the LB Backing Pump OFF?", "Does the EC Backing Pump have a fault?", "Does the LB Backing Pump have a fault?", "Is the EC Backing Pipe at Atmospheric Pressure", "Is the LB Backing Pipe at Atmospheric Pressure", "Is the EC Backing Manifold at Atmospheric Pressure", "s the LB Backing Manifold at Atmospheric Pressure?", "Is the EC Roughing Pipe at Atmospheric Pressure", "Is the LB Roughing Pipe at Atmospheric Pressure?", "Is the EC Roughing Manifold at Atmospheric Pressure", "Is the LB Roughing Manifold at Atmospheric Pressure", "Is LB Backing Manifold Valve Opened?", "Is EC Backing Manifold Valve Opened?", "Is LB Roughing Manifold Valve Opened?", "Is EC Roughing Manifold Valve Opened?", "Is COMP Roughing Valve Opened?", "Is M123 Roughing Valve Opened?", "Is M123 Roughing Valve Closed?", "Is OAP Roughing Valve Opened?", "Is OAP Roughing Valve Closed?", "Is HPBD Roughing Valve Opened?", "Is HPBD Roughing Valve Closed?", "Is BTL Roughing Valve Opened?", "Is BTL Roughing Valve Closed?", "Is TARGET Roughing Valve Opened?", "Is TARGET Roughing Valve Closed?", "Is BTL2 Roughing Valve Opened?", "Is BTL2 Roughing Valve Closed?", "Is HPD Roughing Valve Opened?", "Is HPD Roughing Valve Closed?", "Is COMP Turbo Backing Valve Opened?", "Is M123 Turbo Backing Valve Opened", "Is HPBD Turbo Backing Valve Opened?", "Is OAP Turbo Backing Valve Opened?", "Is BTL Turbo Backing Valve Opened?", "Is TARGET1 Turbo Backing Valve Opened?", "Is TARGET2 Turbo Backing Valve Opened?", "Is BTL2 Turbo Backing Valve Opened?", "Is HPD Turbo Backing Valve Opened?", "Is M123 Backing at MID-VAC?", "Is OAP Backing at MID-VAC?", "Is TARGET1 Backing at MID-VAC?", "Is TARGET2 Backing at MID-VAC?", "Is BTL Backing at MID-VAC?", "Is BTL2 Backing at MID-VAC?", "Is HPD Backing at MID-VAC?", "Is M123 Turbo in Normal Operation", "Is COMP Turbo in Normal Operation", "Is OAP Turbo in Normal Operation", "Is BTL Turbo in Normal Operation", "Is TARGET1 Turbo in Normal Operation", "Is TARGET2 Turbo in Normal Operation", "Is BTL2 Turbo in Normal Operation", "Is HPD Turbo in Normal Operation", "Is M123 at MID-VAC?", "Is OAP at MID-VAC?", "Is COMP at MID-VAC?", "Is BTL at MID-VAC?", "Is TARGET at MID-VAC?", "Is BTL2 at MID-VAC?", "Is HPD at MID-VAC?"]
          }
          frame "BTL" {
            w1633 = T32[] [enum."Is BLT at Atmospheric Pressure", enum."Is the EC Roughing Manifold at Atmospheric Pressure"] items=["No Action", "Is EC GPM Mode ON?", "Is EC GPM Mode Off?", "Is EC GVM Mode ON?", "Is EC GVM Off?", "Is  EC GPM or GVM Mode ON?", "Is LB GPM Mode ON?", "Is LB GPM Mode Off?", "Is LB GVM Mode ON?", "Is LB GVM Mode Off?", "Is  LB GPM or GVM Mode ON?", "Is M123 Turbo Gate Valve Opened? ", "Is M123 Turbo Gate Valve Closed?", "Is OAP Turbo Gate Valve Opened?", "Is OAP Turbo Gate Valve Closed?", "Is BTLTurbo Gate Valve Opened?", "Is BTL Turbo Gate Valve Closed?", "Is TARGET Turbo Gate Valve 1Opened?", "Is TARGET1 Turbo Gate Valve Closed?", "Is TARGET Turbo Gate Valve 2 Opened?", "Is TAREGT2 Turbo Gate Valve Closed?", "Is BTL2 Turbo Gate Valve Opened?", "Is BTL2 Turbo Gate Valve Closed?", "Is HPD Turbo Gate Valve Opened?", "Is HPD Turbo Gate Valve Closed?", "Is COMP to M123 gate Valve Opened?", "Is COMP to M123 Valve Closed?", "Is HPBD Gate Valve Opened?", "Is HPBD Gate Valve Closed?", "Is M123 to OAP gate valve opened?", "Is M123 to OAP gate valve closed?", "Is OAP to BLT gate valve opened?", "Is OAP to BTL Gate Valve Closed?", "Is BLT to TARGET gate valve opened?", "Is BTL to TARGET Gate Valve Closed?", "Is TARGET to BLT2 gate valve opened?", "Is TARGET to BTL2 Gate Valve Closed?", "Is BLT2 to HPD gate valve opened?", "Is BTL2 to HPD Gate Valve Closed?", "Is COMP at Atmospheric Pressure?", "Is M123 at Atmospheric Pressure?", "Is BeamDump at Atmospheric Pressure?", "Is OAP at Atmospheric Pressure?", "Is BLT at Atmospheric Pressure", "Is TARGET at Atmospheric Pressure?", "Is BLT2 at Atmospheric Pressure?", "Is HPD at Atmospheric Pressure?", "Is the EC Roughing Pump ON?", "Is the EC Roughing Pump OFF?", "Does the EC Roughing Pump have a fault?", "Is the LB Roughing Pump ON?", "Is the LB Roughing Pump Off?", "Does the LB Roughing Pump have a fault?", "Is the EC Backing Pump ON?", "Is the EC Backing Pump OFF?", "Is the LB Backing Pump ON?", "Is the LB Backing Pump OFF?", "Does the EC Backing Pump have a fault?", "Does the LB Backing Pump have a fault?", "Is the EC Backing Pipe at Atmospheric Pressure", "Is the LB Backing Pipe at Atmospheric Pressure", "Is the EC Backing Manifold at Atmospheric Pressure", "s the LB Backing Manifold at Atmospheric Pressure?", "Is the EC Roughing Pipe at Atmospheric Pressure", "Is the LB Roughing Pipe at Atmospheric Pressure?", "Is the EC Roughing Manifold at Atmospheric Pressure", "Is the LB Roughing Manifold at Atmospheric Pressure", "Is LB Backing Manifold Valve Opened?", "Is EC Backing Manifold Valve Opened?", "Is LB Roughing Manifold Valve Opened?", "Is EC Roughing Manifold Valve Opened?", "Is COMP Roughing Valve Opened?", "Is M123 Roughing Valve Opened?", "Is M123 Roughing Valve Closed?", "Is OAP Roughing Valve Opened?", "Is OAP Roughing Valve Closed?", "Is HPBD Roughing Valve Opened?", "Is HPBD Roughing Valve Closed?", "Is BTL Roughing Valve Opened?", "Is BTL Roughing Valve Closed?", "Is TARGET Roughing Valve Opened?", "Is TARGET Roughing Valve Closed?", "Is BTL2 Roughing Valve Opened?", "Is BTL2 Roughing Valve Closed?", "Is HPD Roughing Valve Opened?", "Is HPD Roughing Valve Closed?", "Is COMP Turbo Backing Valve Opened?", "Is M123 Turbo Backing Valve Opened", "Is HPBD Turbo Backing Valve Opened?", "Is OAP Turbo Backing Valve Opened?", "Is BTL Turbo Backing Valve Opened?", "Is TARGET1 Turbo Backing Valve Opened?", "Is TARGET2 Turbo Backing Valve Opened?", "Is BTL2 Turbo Backing Valve Opened?", "Is HPD Turbo Backing Valve Opened?", "Is M123 Backing at MID-VAC?", "Is OAP Backing at MID-VAC?", "Is TARGET1 Backing at MID-VAC?", "Is TARGET2 Backing at MID-VAC?", "Is BTL Backing at MID-VAC?", "Is BTL2 Backing at MID-VAC?", "Is HPD Backing at MID-VAC?", "Is M123 Turbo in Normal Operation", "Is COMP Turbo in Normal Operation", "Is OAP Turbo in Normal Operation", "Is BTL Turbo in Normal Operation", "Is TARGET1 Turbo in Normal Operation", "Is TARGET2 Turbo in Normal Operation", "Is BTL2 Turbo in Normal Operation", "Is HPD Turbo in Normal Operation", "Is M123 at MID-VAC?", "Is OAP at MID-VAC?", "Is COMP at MID-VAC?", "Is BTL at MID-VAC?", "Is TARGET at MID-VAC?", "Is BTL2 at MID-VAC?", "Is HPD at MID-VAC?"]
          }
          frame "TARGET" {
            w1634 = T32[] [enum."Is TARGET at Atmospheric Pressure?", enum."Is the EC Roughing Manifold at Atmospheric Pressure"] items=["No Action", "Is EC GPM Mode ON?", "Is EC GPM Mode Off?", "Is EC GVM Mode ON?", "Is EC GVM Off?", "Is  EC GPM or GVM Mode ON?", "Is LB GPM Mode ON?", "Is LB GPM Mode Off?", "Is LB GVM Mode ON?", "Is LB GVM Mode Off?", "Is  LB GPM or GVM Mode ON?", "Is M123 Turbo Gate Valve Opened? ", "Is M123 Turbo Gate Valve Closed?", "Is OAP Turbo Gate Valve Opened?", "Is OAP Turbo Gate Valve Closed?", "Is BTLTurbo Gate Valve Opened?", "Is BTL Turbo Gate Valve Closed?", "Is TARGET Turbo Gate Valve 1Opened?", "Is TARGET1 Turbo Gate Valve Closed?", "Is TARGET Turbo Gate Valve 2 Opened?", "Is TAREGT2 Turbo Gate Valve Closed?", "Is BTL2 Turbo Gate Valve Opened?", "Is BTL2 Turbo Gate Valve Closed?", "Is HPD Turbo Gate Valve Opened?", "Is HPD Turbo Gate Valve Closed?", "Is COMP to M123 gate Valve Opened?", "Is COMP to M123 Valve Closed?", "Is HPBD Gate Valve Opened?", "Is HPBD Gate Valve Closed?", "Is M123 to OAP gate valve opened?", "Is M123 to OAP gate valve closed?", "Is OAP to BLT gate valve opened?", "Is OAP to BTL Gate Valve Closed?", "Is BLT to TARGET gate valve opened?", "Is BTL to TARGET Gate Valve Closed?", "Is TARGET to BLT2 gate valve opened?", "Is TARGET to BTL2 Gate Valve Closed?", "Is BLT2 to HPD gate valve opened?", "Is BTL2 to HPD Gate Valve Closed?", "Is COMP at Atmospheric Pressure?", "Is M123 at Atmospheric Pressure?", "Is BeamDump at Atmospheric Pressure?", "Is OAP at Atmospheric Pressure?", "Is BLT at Atmospheric Pressure", "Is TARGET at Atmospheric Pressure?", "Is BLT2 at Atmospheric Pressure?", "Is HPD at Atmospheric Pressure?", "Is the EC Roughing Pump ON?", "Is the EC Roughing Pump OFF?", "Does the EC Roughing Pump have a fault?", "Is the LB Roughing Pump ON?", "Is the LB Roughing Pump Off?", "Does the LB Roughing Pump have a fault?", "Is the EC Backing Pump ON?", "Is the EC Backing Pump OFF?", "Is the LB Backing Pump ON?", "Is the LB Backing Pump OFF?", "Does the EC Backing Pump have a fault?", "Does the LB Backing Pump have a fault?", "Is the EC Backing Pipe at Atmospheric Pressure", "Is the LB Backing Pipe at Atmospheric Pressure", "Is the EC Backing Manifold at Atmospheric Pressure", "s the LB Backing Manifold at Atmospheric Pressure?", "Is the EC Roughing Pipe at Atmospheric Pressure", "Is the LB Roughing Pipe at Atmospheric Pressure?", "Is the EC Roughing Manifold at Atmospheric Pressure", "Is the LB Roughing Manifold at Atmospheric Pressure", "Is LB Backing Manifold Valve Opened?", "Is EC Backing Manifold Valve Opened?", "Is LB Roughing Manifold Valve Opened?", "Is EC Roughing Manifold Valve Opened?", "Is COMP Roughing Valve Opened?", "Is M123 Roughing Valve Opened?", "Is M123 Roughing Valve Closed?", "Is OAP Roughing Valve Opened?", "Is OAP Roughing Valve Closed?", "Is HPBD Roughing Valve Opened?", "Is HPBD Roughing Valve Closed?", "Is BTL Roughing Valve Opened?", "Is BTL Roughing Valve Closed?", "Is TARGET Roughing Valve Opened?", "Is TARGET Roughing Valve Closed?", "Is BTL2 Roughing Valve Opened?", "Is BTL2 Roughing Valve Closed?", "Is HPD Roughing Valve Opened?", "Is HPD Roughing Valve Closed?", "Is COMP Turbo Backing Valve Opened?", "Is M123 Turbo Backing Valve Opened", "Is HPBD Turbo Backing Valve Opened?", "Is OAP Turbo Backing Valve Opened?", "Is BTL Turbo Backing Valve Opened?", "Is TARGET1 Turbo Backing Valve Opened?", "Is TARGET2 Turbo Backing Valve Opened?", "Is BTL2 Turbo Backing Valve Opened?", "Is HPD Turbo Backing Valve Opened?", "Is M123 Backing at MID-VAC?", "Is OAP Backing at MID-VAC?", "Is TARGET1 Backing at MID-VAC?", "Is TARGET2 Backing at MID-VAC?", "Is BTL Backing at MID-VAC?", "Is BTL2 Backing at MID-VAC?", "Is HPD Backing at MID-VAC?", "Is M123 Turbo in Normal Operation", "Is COMP Turbo in Normal Operation", "Is OAP Turbo in Normal Operation", "Is BTL Turbo in Normal Operation", "Is TARGET1 Turbo in Normal Operation", "Is TARGET2 Turbo in Normal Operation", "Is BTL2 Turbo in Normal Operation", "Is HPD Turbo in Normal Operation", "Is M123 at MID-VAC?", "Is OAP at MID-VAC?", "Is COMP at MID-VAC?", "Is BTL at MID-VAC?", "Is TARGET at MID-VAC?", "Is BTL2 at MID-VAC?", "Is HPD at MID-VAC?"]
          }
          frame "BTL2" {
